vi "Launch Connection Factory.vi"(8 "error in (no error)":errorcluster, 11 "MultiplexedConnectionHandler in":refnum<class "MultiplexedConnectionHandler.lvclass">) -> (0 "error out":errorcluster, 3 "MultiplexedConnectionHandler out":refnum<class "MultiplexedConnectionHandler.lvclass">)   [LabVIEW 2020, in "MultiplexedConnectionHandler.lvlib" / "MultiplexedConnectionHandler.lvclass"]
uses:
  <vilib>/gpm_packages/@cs/Network-interface/Source/MultiplexedConnectionHandler/MultiplexedConnectionHandler/MultiplexedConnectionHandler.lvclass
  C:/Program Files/National Instruments/LabVIEW 2020/vi.lib/gpm_packages/@cs/Network-interface/Source/PersistantConnectionHandler/PersistantConnectionHandler/PersistantConnectionHandler.lvclass
  <vilib>/gpm_packages/@cs/Network-interface/Source/MultiplexedConnectionHandler/MultiplexedConnectionHandler/MultiplexedConnectionHandler.lvclass/MultiplexedConnectionHandler.ctl
  <vilib>/gpm_packages/@cs/Network-interface/Source/PersistantConnectionHandler/PersistantConnectionHandler/PersistantConnectionHandler.lvclass
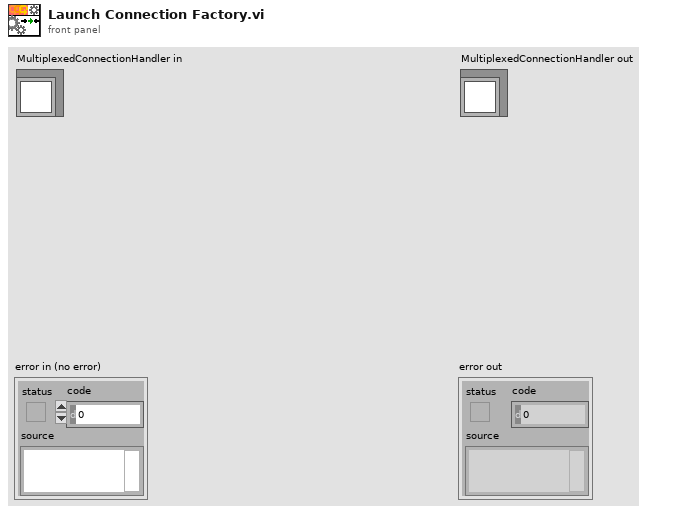
[diagram p1: front panel]
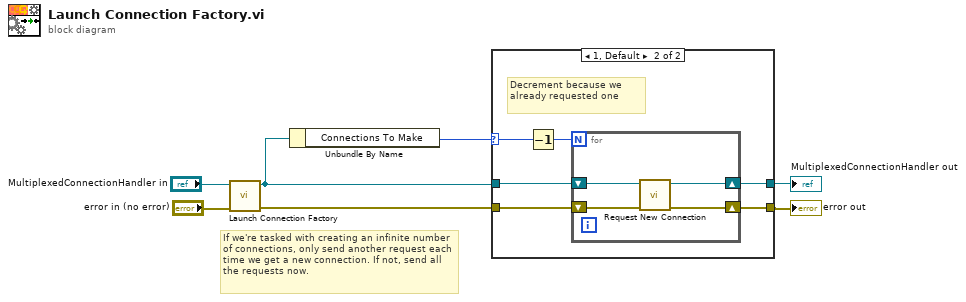
[diagram p0: block diagram]
diagram:
  # "If we're tasked with creating an infinite number of connections, only send another request each time we get a new connection. If not, send all the requests now."
  n1 = call-parent "Launch Connection Factory.vi"("error in (no error)"="error in (no error)", "PersistantConnectionHandler in"="MultiplexedConnectionHandler in") -> ("error out"=w5:errorcluster, "PersistantConnectionHandler out"=w4:refnum<class "MultiplexedConnectionHandler.lvclass">)  [unwired: 8 in]
  n2 = Unbundle By Name(w4) -> ("Connections To Make"=w3:i32)
  n3 = case shown="1, Default" w3 {
    selector: w3 -> [_ w10]
    tunnel: w4 -> [w9 w15]
    tunnel: w5 -> [w8 w14]
    tunnel: [w9 w13] -> w2
    tunnel: [w8 w12] -> w1
    frame -1 {
    }
    frame 1, Default {
      # "Decrement because we already requested one"
      n4 = Decrement(x=w10) -> (x-1=w11:i32)
      n5 = for {
        N: w11 -> [_]
        shift-right: [w18] -> w13
        shift-left: w15 -> [w19]
        shift-right: [w16] -> w12
        shift-left: w14 -> [w17]
        n6 = call <vilib>:"Request New Connection.vi"("error in (no error)"=w17, "PersistantConnectionHandler in"=w19) -> ("error out"=w16:errorcluster, "PersistantConnectionHandler out"=w18:refnum<class "MultiplexedConnectionHandler.lvclass">)  [unwired: 8 in]
      }
    }
  }
  "error out" <- w1
  "MultiplexedConnectionHandler out" <- w2
